vi "Write States.vi"(8 "error in (no error)":errorcluster, 10 "States":enum16{"Halt", "Exit", "GoTo"}(ring), 11 "TableReceiverTactic in":refnum<class "TableReceiverTactic.lvclass">) -> (0 "error out":errorcluster, 3 "TableReceiverTactic out":refnum<class "TableReceiverTactic.lvclass">)   [LabVIEW 2023, in "TableReceiverTactic.lvclass"]
uses:
  TableReceiverTactic.lvclass
  TableReceiverTactic.lvclass/TableReceiverTactic.ctl
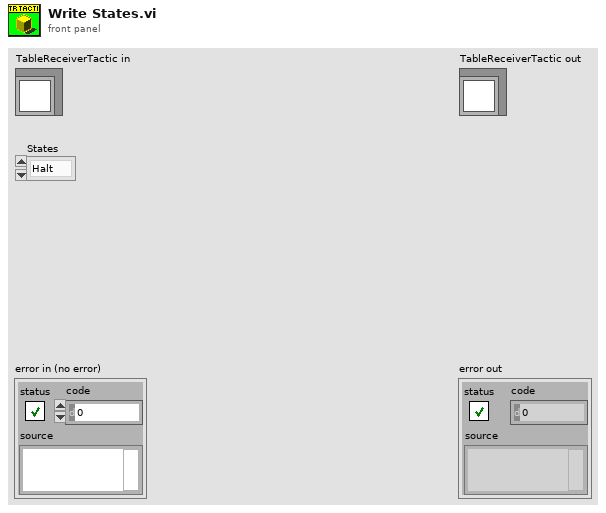
[diagram p1: front panel]
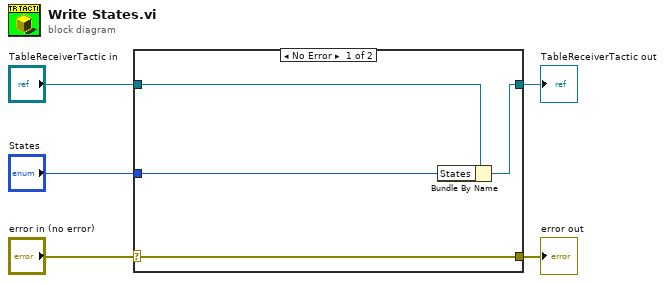
[diagram p0: block diagram]
diagram:
  n1 = case shown="No Error" "error in (no error)" {
    selector: "error in (no error)" -> [w9 w10]
    tunnel: [w9 w10] -> w4
    tunnel: [w7 w11] -> w2
    tunnel: "TableReceiverTactic in" -> [w8 w11]
    tunnel: "States" -> [w6 _]
    frame No Error {
      n2 = Bundle By Name(cluster=w8, "States"=w6) -> (w7:refnum<class "TableReceiverTactic.lvclass">)
    }
    frame Error {
    }
  }
  "error out" <- w4
  "TableReceiverTactic out" <- w2
